vi "Reference to Waveform.vi"(5 "Data":refnum<data-value>, 12 "error in (no error)":errorcluster) -> (6 "Waveform":cluster{"t0":dbl, "dt":dbl, "y":csg[]}, 14 "error out":errorcluster)   [LabVIEW 2016, in "Common.lvlib"]
uses:
  Common.lvlib
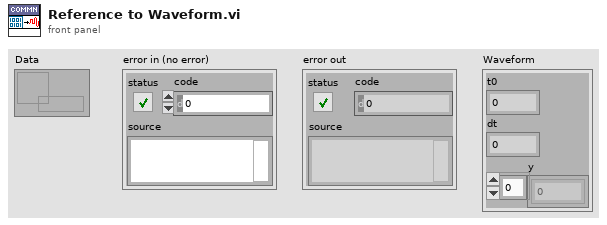
[diagram p1: front panel]
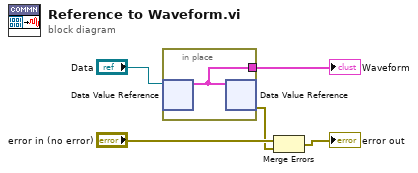
[diagram p0: block diagram]
diagram:
  n1 = in-place {
    in-place-border: [w6] -> w1
    n2 = in-place-dvr #1("Data") -> (w6:cluster{"t0":dbl, "dt":dbl, "y":csg[]})  [unwired: 1 out]
    n3 = in-place-dvr #1(w6) -> (w2:errorcluster)  [unwired: 1 out]
  }
  "Waveform" <- w1
  n4 = Merge Errors("error in (no error)", w2) -> (→"error out":errorcluster)
